vi "JSON Action Data to String Data.vi"(8 "error in (no error)":errorcluster, 9 "Action Data (JSON)":string, 10 "data type":enum16{"INT", "DBL", "BOOL", "String"}(ring), 11 "path":string) -> (0 "error out":errorcluster, 3 "String":string)   [LabVIEW 2016, in "Hardware.lvlib" / "Motions.lvlib" / "Motions.lvclass"]
uses:
  <userlib>/Common Components/Hardware/Abstract System/Motions/Motions/Motions.lvclass
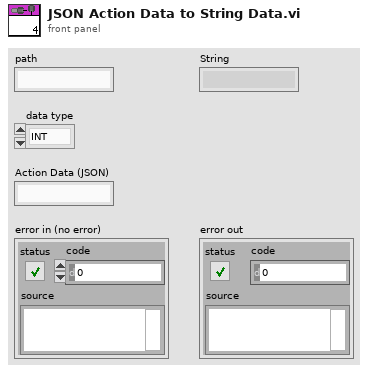
[diagram p1: front panel]
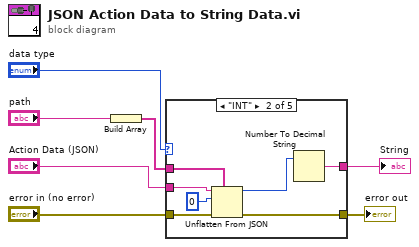
[diagram p0: block diagram]
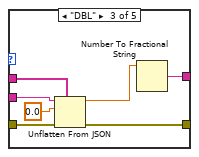
[diagram p3: hidden frame]
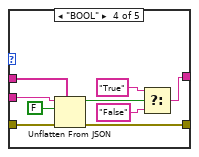
[diagram p4: hidden frame]
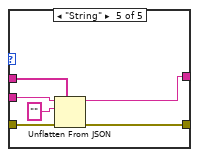
[diagram p5: hidden frame]
diagram:
  n1 = Build Array("path") -> (w1:string[])
  n2 = case shown="\"INT\"" "data type" {
    tunnel: "Action Data (JSON)" -> [_ w15 w21 w31 w37]
    tunnel: w1 -> [_ w9 w16 w23 w32]
    tunnel: [_ w12 w19 w26 w35] -> w5
    tunnel: "error in (no error)" -> [w8 w11 w18 w25 w34]
    tunnel: [w8 w10 w17 w24 w33] -> w7
    frame Default {
    }
    frame "INT" {
      n3 = Unflatten From JSON(path=w9, JSON string=w15, type and defaults=0, error in (no error)=w11) -> (value=w13:i32, error out=w10:errorcluster)  [unwired: 3 in]
      n4 = Number To Decimal String(number=w13) -> (decimal integer string=w12:string)  [unwired: 1 in]
    }
    frame "DBL" {
      n5 = Unflatten From JSON(path=w16, JSON string=w21, type and defaults=0.0, error in (no error)=w18) -> (value=w22:dbl, error out=w17:errorcluster)  [unwired: 3 in]
      n6 = Number To Fractional String(number=w22) -> (F-format string=w19:string)  [unwired: 3 in]
    }
    frame "BOOL" {
      n7 = Unflatten From JSON(path=w23, JSON string=w31, type and defaults=FALSE, error in (no error)=w25) -> (value=w29:bool, error out=w24:errorcluster)  [unwired: 3 in]
      n8 = Select(t="True", s=w29, f="False") -> (s? t:f=w26:string)
    }
    frame "String" {
      n9 = Unflatten From JSON(path=w32, JSON string=w37, type and defaults="", error in (no error)=w34) -> (value=w35:string, error out=w33:errorcluster)  [unwired: 3 in]
    }
  }
  "error out" <- w7
  "String" <- w5
